vi "generatestitchingmacroforfiji.vi"(11 "file":path) -> ()   [LabVIEW 2012]
doc: "SciScan 1.2 160622"
uses:
  GFG/GFGnumericGet.vi
  GFG/GFGbooleanGet.vi
  GFG/GFG library.lvlib
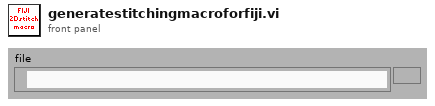
[diagram p1: front panel]
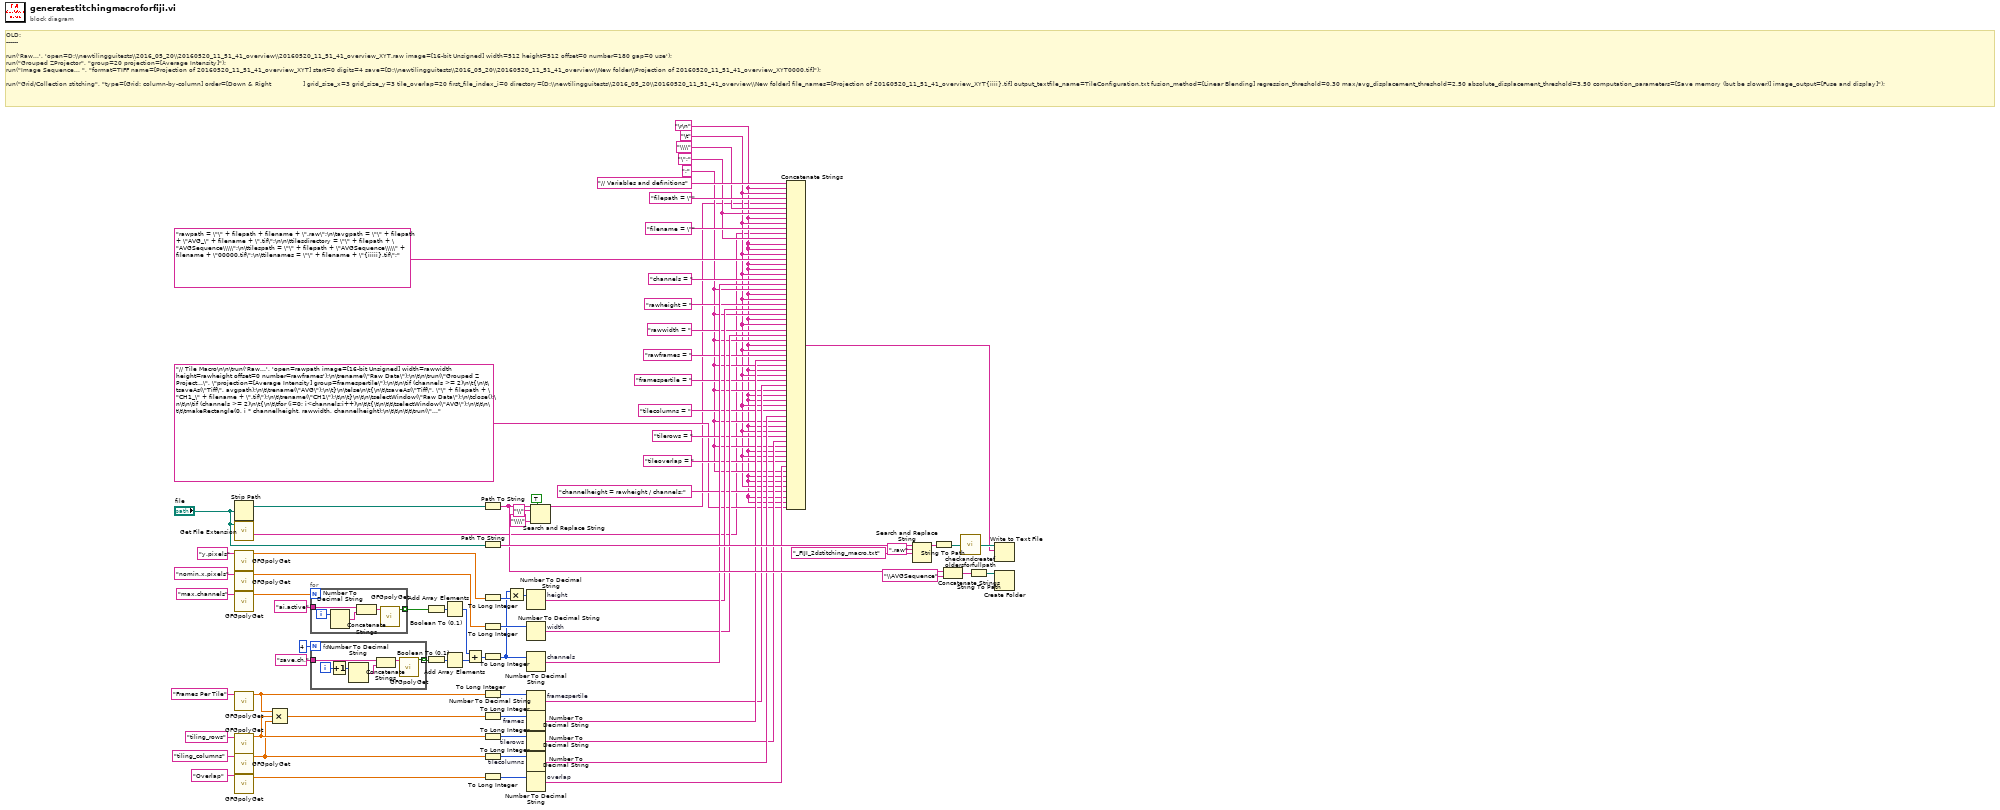
[diagram p0: block diagram]
diagram:
  w43 = "\";" ("string")
  w10 = ";" ("string")
  w9 = "\t"
  w7 = "\r\n"
  # "OLD:\n------\n\nrun('Raw...', 'open=D:\\\\newtilingguitests\\\\2016_05_20\\\\20160520_11_51_41_overview\\\\20160520_11_51_41_overview_XYT.raw image=[16-bit Unsigned] width=512 height=512 offset=0 number=180 gap=0 use');\nrun(\"Grouped ZProjector\", \"group=20 projection=[Average Intensity]\");\nrun(\"Image Sequence... \", \"format=TIFF name=[Projection of 20160520_11_51_41_overview_XYT] start=0 digits=4 save=[D:\\\\newtilingguitests\\\\2016_05_20\\\\20160520_11_51_41_overview\\\\New folder\\\\Projection of 20160520_11_51_41_overview_XYT0000.tif]\");\n\nrun(\"Grid/Collection stitching\", \"type=[Grid: column-by-column] order=[Down & Right                ] grid_size_x=3 grid_size_y=3 tile_overlap=20 first_file_index_i=0 directory=[D:\\\\newtilingguitests\\\\2016_05_20\\\\20160520_11_51_41_overview\\\\New folder] file_names=[Projection of 20160520_11_51_41_overview_XYT{iiii}.tif] output_textfile_name=TileConfiguration.txt fusion_method=[Linear Blending] regression_threshold=0.30 max/avg_displacement_threshold=2.50 absolute_displacement_threshold=3.50 computation_parameters=[Save memory (but be slower)] image_output=[Fuse and display]\");"
  n1 = Strip Path(path="file") -> (stripped path=w70:path)  [unwired: 1 out]
  n2 = call <vilib>:"Get File Extension.vi"("file"="file") -> ("filename without extension"=w4:string)  [unwired: 7 in, 3 out]
  n3 = call-poly "GFGpolyGet.vi"("Variable Name in"="y.pixels") -> ("Numeric"=w38:dbl)  [unwired: 8 in, 2 out]
  n4 = call-poly "GFGpolyGet.vi"("Variable Name in"="nomin.x.pixels") -> ("Numeric"=w40:dbl)  [unwired: 8 in, 2 out]
  n5 = call-poly "GFGpolyGet.vi"("Variable Name in"="max.channels") -> ("Numeric"=w61:dbl)  [unwired: 8 in, 2 out]
  n6 = call-poly "GFGpolyGet.vi"("Variable Name in"="Frames Per Tile") -> ("Numeric"=w26:dbl)  [unwired: 8 in, 2 out]
  n7 = call-poly "GFGpolyGet.vi"("Variable Name in"="tiling_rows") -> ("Numeric"=w24:dbl)  [unwired: 8 in, 2 out]
  n8 = call-poly "GFGpolyGet.vi"("Variable Name in"="tiling_columns") -> ("Numeric"=w22:dbl)  [unwired: 8 in, 2 out]
  n9 = call-poly "GFGpolyGet.vi"("Variable Name in"="Overlap") -> ("Numeric"=w1:dbl)  [unwired: 8 in, 2 out]
  n10 = Compound Arithmetic op=MULTIPLY(w26, w24, w22) -> (w3:dbl)
  n11 = for {
    N: w61 -> [_]
    tunnel: [w84] -> w63 mode=indexing
    tunnel: "ai.active" ("Variable Name in") -> [w83]
    i -> [w82]
    n12 = Number To Decimal String(number=w82) -> (decimal integer string=w81:string)  [unwired: 1 in]
    n13 = Concatenate Strings(w83, w81) -> (w80:string)
    n14 = call-poly "GFGpolyGet.vi"("Variable Name in"=w80) -> ("Boolean Value OUT"=w84:bool)  [unwired: 9 in, 1 out]
  }
  n15 = for {
    N: 4 -> [_]
    tunnel: "save.ch." ("Variable Name in") -> [w90]
    tunnel: [w89] -> w57 mode=indexing
    i -> [w88]
    n16 = Increment(x=w88) -> (x+1=w87:i32)
    n17 = Number To Decimal String(number=w87) -> (decimal integer string=w85:string)  [unwired: 1 in]
    n18 = Concatenate Strings(w90, w85) -> (w86:string)
    n19 = call-poly "GFGpolyGet.vi"("Variable Name in"=w86) -> ("Boolean Value OUT"=w89:bool)  [unwired: 9 in, 1 out]
  }
  n20 = Boolean To (0,1)(Boolean=w63) -> (0, 1=w64:i16[])
  n21 = Boolean To (0,1)(Boolean=w57) -> (0, 1=w58:i16[])
  n22 = Add Array Elements(numeric array=w64) -> (sum=w55:i16)
  n23 = Add Array Elements(numeric array=w58) -> (sum=w54:i16)
  n24 = Add(x=w55, y=w54) -> (x+y=w36:i16)
  n25 = Path To String(path=w70) -> (string=w46:string)
  n26 = Path To String(path="file") -> (string=w69:string)
  n27 = To Long Integer(number=w38) -> (32bit integer=w37:i32)
  n28 = To Long Integer(number=w40) -> (32bit integer=w39:i32)
  n29 = To Long Integer(number=w36) -> (32bit integer=w34:i32)
  n30 = To Long Integer(number=w26) -> (32bit integer=w25:i32)
  n31 = To Long Integer(number=w3) -> (32bit integer=w27:i32)
  n32 = To Long Integer(number=w24) -> (32bit integer=w23:i32)
  n33 = To Long Integer(number=w22) -> (32bit integer=w21:i32)
  n34 = To Long Integer(number=w1) -> (32bit integer=w12:i32)
  n35 = Multiply(x=w34, y=w37) -> (x*y=w35:i32)
  n36 = Number To Decimal String "height"(number=w35) -> (decimal integer string=w31:string)  [unwired: 1 in]
  n37 = Number To Decimal String "width"(number=w39) -> (decimal integer string=w29:string)  [unwired: 1 in]
  n38 = Number To Decimal String "channels"(number=w34) -> (decimal integer string=w33:string)  [unwired: 1 in]
  n39 = Number To Decimal String "framespertile"(number=w25) -> (decimal integer string=w18:string)  [unwired: 1 in]
  n40 = Number To Decimal String "frames"(number=w27) -> (decimal integer string=w20:string)  [unwired: 1 in]
  n41 = Number To Decimal String "tilerows"(number=w23) -> (decimal integer string=w14:string)  [unwired: 1 in]
  n42 = Number To Decimal String "tilecolumns"(number=w21) -> (decimal integer string=w16:string)  [unwired: 1 in]
  n43 = Number To Decimal String "overlap"(number=w12) -> (decimal integer string=w11:string)  [unwired: 1 in]
  n44 = Search and Replace String(replace all?=TRUE ("replace all? (F)"), input string=w46, search string="\\", replace string="\\\\" ("replace string (\"\")")) -> (result string=w2:string)  [unwired: 4 in, 3 out]
  n45 = Concatenate Strings("// Variables and definitions" ("string"), w7, w9, "filepath = \"" ("string"), w2, "\\\\" ("string"), w43, w7, w9, "filename = \"" ("string"), w4, w43, w7, w7, w9, "rawpath = \"\" + filepath + filename + \".raw\";\n\tavgpath = \"\" + filepath + \"AVG_\" + filename + \".tif\";\n\n\ttilesdirectory = \"\" + filepath + \"AVGSequence\\\\\";\n\ttilespath = \"\" + filepath + \"AVGSequence\\\\\" + filename + \"00000.tif\";\n\ttilenames = \"\" + filename + \"{iiiii}.tif\";" ("string"), w7, w7, w9, "channels = " ("string"), w33, w10, w7, w9, "rawheight = " ("string"), w31, w10, w7, w9, "rawwidth = " ("string"), w29, w10, w7, w9, "rawframes = " ("string"), w20, w10, w7, w9, "framespertile = " ("string"), w18, w10, w7, w7, w9, "tilecolumns = " ("string"), w16, w10, w7, w9, "tilerows = " ("string"), w14, w10, w7, w9, "tileoverlap = " ("string"), w11, w10, w7, w7, w9, "channelheight = rawheight / channels;" ("string"), w7, w7, "// Tile Macro\n\n\trun('Raw...', 'open=rawpath image=[16-bit Unsigned] width=rawwidth height=rawheight offset=0 number=rawframes');\n\trename(\"Raw Data\");\n\t\n\trun(\"Grouped Z Project...\", \"projection=[Average Intensity] group=framespertile\");\n\t\n\tif (channels >= 2)\n\t{\n\t\tsaveAs(\"Tiff\", avgpath);\n\t\trename(\"AVG\");\n\t}\n\telse\n\t{\n\t\tsaveAs(\"Tiff\", \"\" + filepath + \"CH1_\" + filename + \".tif\");\n\t\trename(\"CH1\");\t\n\t}\n\t\n\tselectWindow(\"Raw Data\");\n\tclose();\n\t\n\tif (channels >= 2)\n\t{\n\t\tfor (i=0; i<channels;i++)\n\t\t{\t\n\t\t\tselectWindow(\"AVG\");\n\t\t\n\t\t\tmakeRectangle(0, i * channelheight, rawwidth, channelheight);\n\t\t\n\t\t\trun(\"Crop\");\n\t\t\t\n\t\t\tsaveAs(\"Tiff\", \"\" + filepath + \"CH\" + i+1 + \"_\" + filename + \".tif\");\n\t\t\t\n\t\t\trename(\"CH\" + i+1 + \"\");\n\t\t\t\n\t\t\topen(\"\" + avgpath + \"\");\n\t\t\trename(\"AVG\");\n\t\t}\n\n\t\tselectWindow(\"AVG\");\n\t\tclose();\n\t}\n\telse\n\t{\t\n\t\tselectWindow(\"CH1\");\t\n\t}\n\t\n\tfor (i=0; i<channels;i++)\n\t{\n\t\tselectWindow(\"CH\" + i+1 + \"\");\n\t\n\t\trun(\"Image Sequence... \", \"format=TIFF name=[\" + filename + \"] start=0 digits=5 save=[\" + tilespath + \"]\");\n\t\n\t\trun(\"Grid/Collection stitching\", \"type=[Grid: column-by-column] order=[Down & Right                ] grid_size_x=[\" + tilecolumns +\"] grid_size_y=[\" + tilerows + \"] tile_overlap=[\" + tileoverlap + \"] first_file_index_i=0 directory=[\" + tilesdirectory + \"] file_names=[\" + tilenames + \"] output_textfile_name=TileConfiguration.txt fusion_method=[Linear Blending] regression_threshold=0.30 max/avg_displacement_threshold=2.50 absolute_displacement_threshold=3.50 computation_parameters=[Save memory (but be slower)] image_output=[Fuse and display]\");\t\t\n\t\tsaveAs(\"Tiff\", \"\" + filepath + \"CH\" + i+1 + \"_Fusion_\" + filename + \".tif\");\n\t\t\n\t}\n\n\trun(\"Tile\");" ("string")) -> (w5:string)
  n46 = Search and Replace String(input string=w69, search string=".raw", replace string="_FIJI_2dstitching_macro.txt" ("string")) -> (result string=w77:string)  [unwired: 5 in, 3 out]
  n47 = String To Path(string=w77) -> (path=w75:path)
  n48 = Concatenate Strings(w46, "\\AVGSequence" ("string")) -> (w53:string)
  n49 = call "checkandcreatefoldersforfullpath.vi"("Path IN"=w75) -> ("Path OUT"=w74:path)  [unwired: 4 in]
  n50 = String To Path(string=w53) -> (path=w52:path)
  n51 = Write to Text File(file (use dialog)=w74, text=w5) -> ()  [unwired: 2 in, 3 out]
  n52 = Create Folder(path (use dialog)=w52) -> ()  [unwired: 2 in, 3 out]
